vi "csum_in9fff.vi"(11 "string":string) -> (0 "hex integer string":string, 3 "x+1 2":u8=151 format="%x")   [LabVIEW 2011]
panel:
  out "length":i32
  out "x+1":u32 format="%x"
  out "Numeric 2":u32
  out "latest":string
  out "round loop":i32
  out "mod 2 is 0 or 1":i32
  out "round count":i32
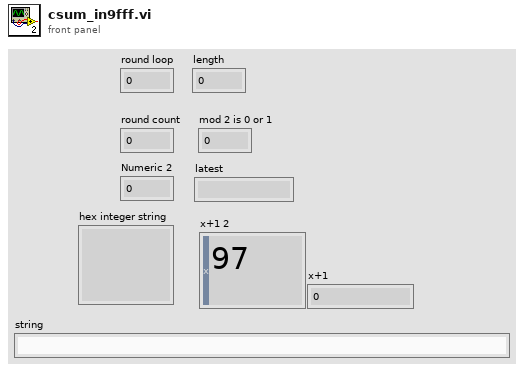
[diagram p1: front panel]
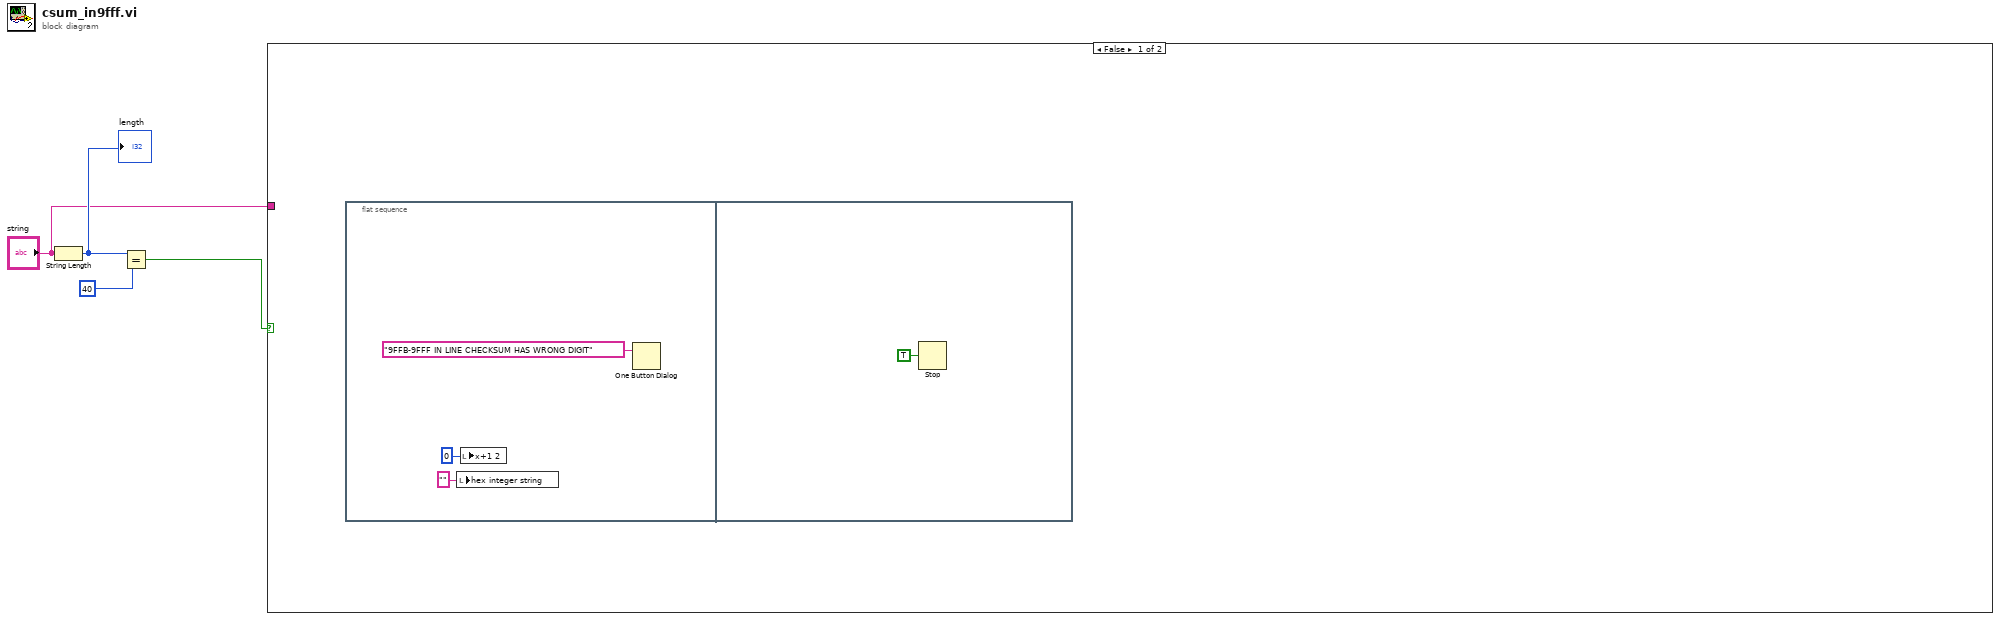
[diagram p0: block diagram]
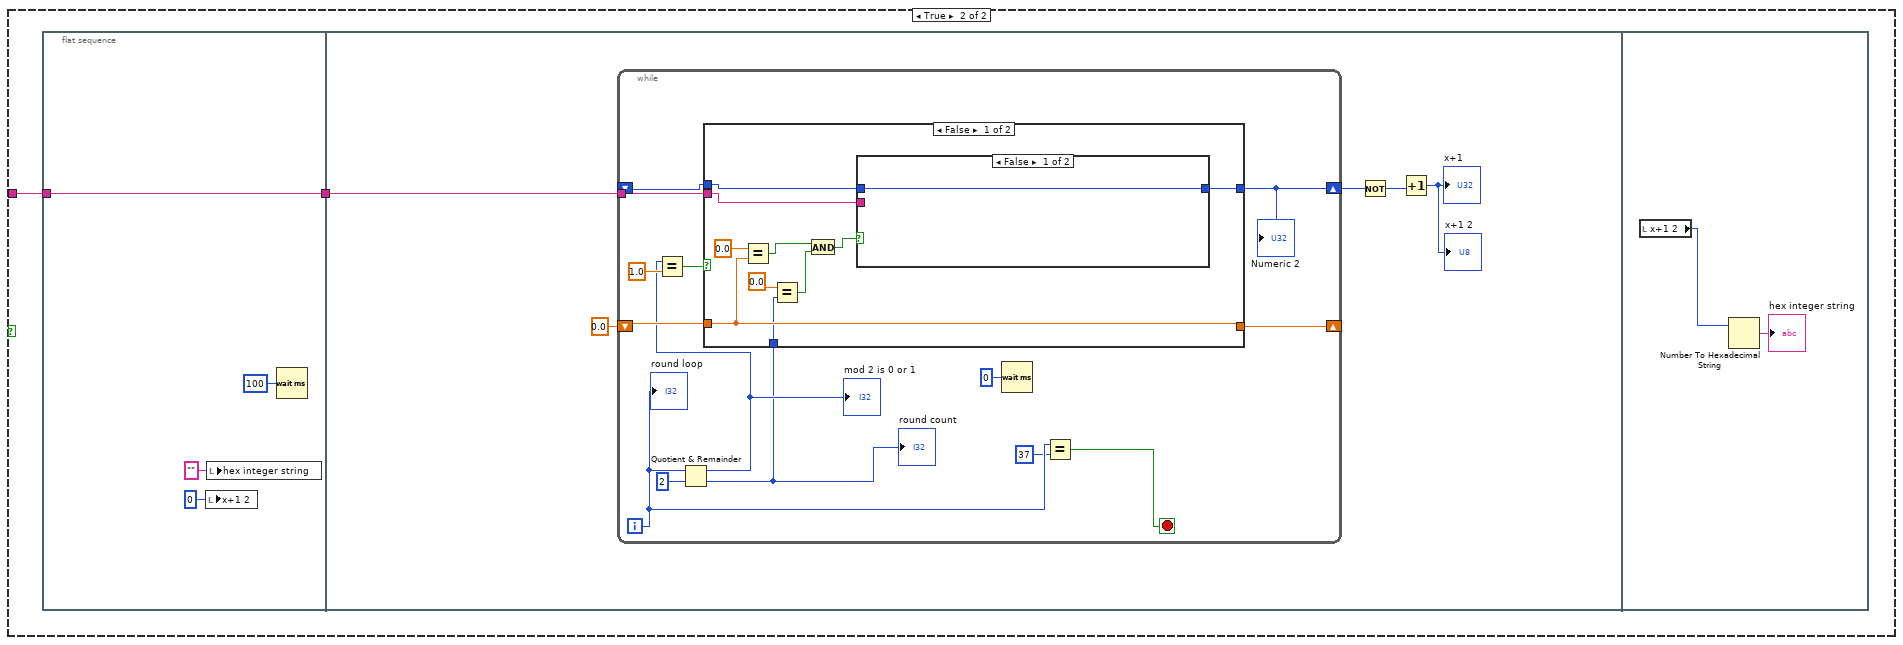
[diagram p2: hidden frame]
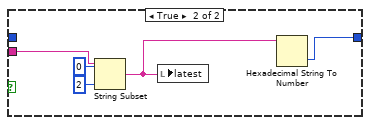
[diagram p3: hidden frame]
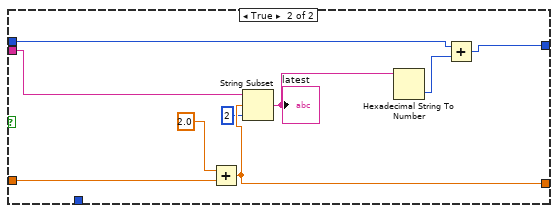
[diagram p4: hidden frame]
diagram:
  n1 = String Length(string="string") -> (length=w3:i32)
  "length" <- w3
  n2 = Equal?(x=w3, y=40) -> (x = y?=w2:bool)
  n3 = case shown="False" w2 {
    tunnel: "string" -> [_ w10]
    frame False {
      n4 = flat-sequence {
        frame #0 {
          n5 = local write "hex integer string"("" ("hex integer string")) -> ()
          n6 = local write "x+1 2"(u8 0 ("x+1 2")) -> ()
          n7 = One Button Dialog(message="9FFB-9FFF IN LINE CHECKSUM HAS WRONG DIGIT") -> ()  [unwired: 1 in, 1 out]
        }
        frame #1 {
          n8 = Stop(stop? (T)=TRUE) -> ()
        }
      }
    }
    frame True {
      n9 = flat-sequence {
        tunnel: w10 -> [w12]
        tunnel: [w12] -> w9
        tunnel: w9 -> [w15]
        frame #0 {
          n10 = local write "x+1 2"(u8 0 ("x+1 2")) -> ()
          n11 = local write "hex integer string"("" ("hex integer string")) -> ()
          n12 = Wait (ms)(milliseconds to wait=u32 100) -> ()  [unwired: 1 out]
        }
        frame #1 {
          n13 = while {
            shift-right: [w29] -> _
            shift-left: 0.0 -> [w28]
            tunnel: w15 -> [w24]
            shift-right: [w23] -> w18
            shift-left: _ -> [w22]
            i -> [w31]
            stop <- w32 stop-if-true
            n14 = Quotient & Remainder(x=w31, y=2) -> (x-y*floor(x/y)=w25:i32, floor(x/y)=w20:i32)
            "round count" <- w20
            "mod 2 is 0 or 1" <- w25
            n15 = Equal?(x=w25, y=1.0) -> (x = y?=w27:bool)
            n16 = case shown="False" w27 {
              tunnel: [w43 w56] -> w29
              tunnel: w28 -> [w43 w58]
              tunnel: w24 -> [w41 w54]
              tunnel: [w40 w52] -> w23
              tunnel: w22 -> [w39 w51]
              tunnel: w20 -> [w34 _]
              frame False {
                n17 = Equal?(x=0.0, y=w43) -> (x = y?=w37:bool)
                n18 = Equal?(x=0.0, y=w34) -> (x = y?=w36:bool)
                n19 = And(x=w37, y=w36) -> (x .and. y?=w38:bool)
                n20 = case shown="False" w38 {
                  tunnel: w41 -> [_ w48]
                  tunnel: [w44 w45] -> w40
                  tunnel: w39 -> [w44 _]
                  frame False {
                  }
                  frame True {
                    n21 = String Subset(string=w48, offset (0)=0, length (rest)=2 ("length (rest)")) -> (substring=w46:string)
                    n22 = local write "latest"(w46) -> ()
                    n23 = Hexadecimal String To Number(string=w46) -> (number=w45:u32)  [unwired: 2 in, 1 out]
                  }
                }
              }
              frame True {
                n24 = Add(x=2.0, y=w58) -> (x+y=w56:dbl)
                n25 = String Subset(string=w54, offset (0)=w56, length (rest)=2 ("length (rest)")) -> (substring=w50:string)
                "latest" <- w50
                n26 = Hexadecimal String To Number(string=w50) -> (number=w53:u32)  [unwired: 2 in, 1 out]
                n27 = Add(x=w51, y=w53) -> (x+y=w52:u32)
              }
            }
            "Numeric 2" <- w23
            n28 = Wait (ms)(milliseconds to wait=u32 0) -> ()  [unwired: 1 out]
            n29 = Equal?(x=w31, y=37) -> (x = y?=w32:bool)
            "round loop" <- w31
          }
          n30 = Not(x=w18) -> (.not. x?=w17:u32)
          n31 = Increment(x=w17) -> (x+1=→"x+1" →"x+1 2":u32)
        }
        frame #2 {
          n32 = local read "x+1 2"() -> (w59:u8)
          n33 = Number To Hexadecimal String(2:w59) -> (0:→"hex integer string":string)  [unwired: 1 in]
        }
      }
    }
  }
